vi "test_extended_video.vi"() -> ()   [LabVIEW 2023]
uses:
  <vilib>/picture/picture.llb/Draw True-Color Pixmap.vi
panel:
  in  "profile_index":sgl=4.0
  in  "source_index":sgl=2.0
  in  "group_index":sgl
  out "metadata":T1
  in  "host":string="192.168.1.7"
  in  "path in":path=path "C:/Users/jcds/Documents/GitHub/hl2ss/extensions/client_labview/hl2ss_labview/hl2ss_ulm.dll"
  out "Pose":sgl[][](array[numeric])
  out "Video":picture
  in  "stop":bool
  in  "Framerate":u8=30
  in  "Height":u16=360
  in  "Width":u16=640
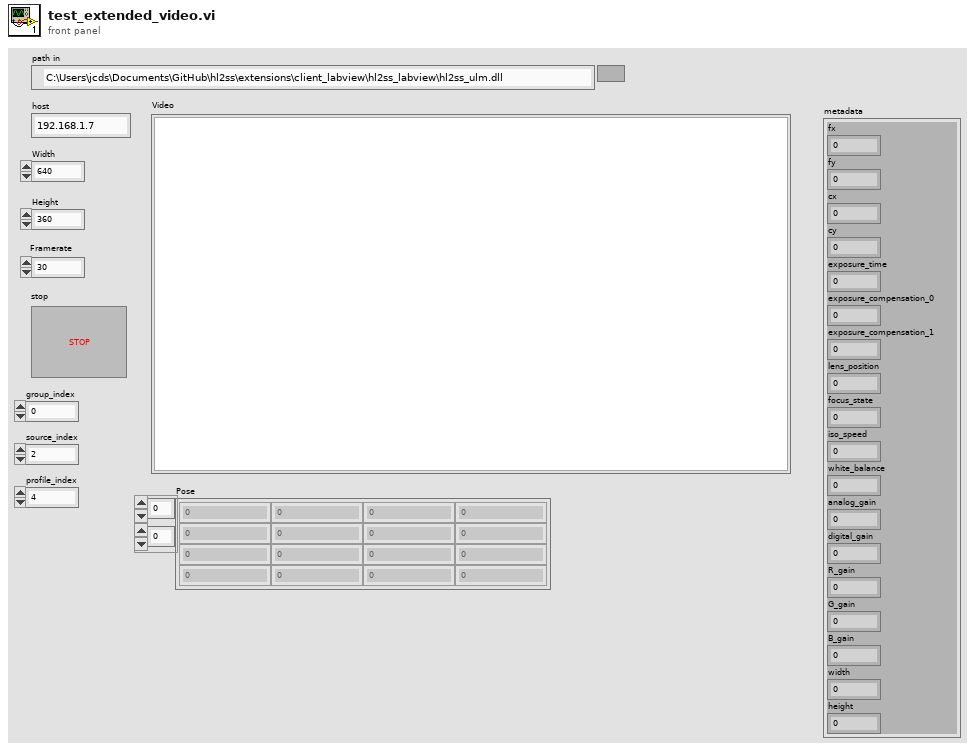
[diagram p1: front panel]
types:
  T1 = cluster{"fx":sgl, "fy":sgl, "cx":sgl, "cy":sgl, "exposure_time":u64, "exposure_compensation_0":u64, "exposure_compensation_1":u64, "lens_position":u32, "focus_state":u32, "iso_speed":u32, "white_balance":u32, "analog_gain":sgl, "digital_gain":sgl, "R_gain":sgl, "G_gain":sgl, "B_gain":sgl, "width":u16, "height":u16}
  T2 = cluster{"enable_mrc":u8, "hologram_composition":u8, "recording_indicator":u8, "video_stabilization":u8, "blank_protected":u8, "show_mesh":u8, "shared":u8, "_reserved_0":u8, "global_opacity":sgl, "output_width":sgl, "output_height":sgl, "video_stabilization_length":u32, "hologram_perspective":u32, "_reserved_1":u32}
  T3 = cluster{"chunk":u64, "mode":u8, "_reserved_0":u8, "width":u16, "height":u16, "framerate":u8, "divisor":u8, "profile":u8, "level":u8, "_reserved_1":u16, "bitrate":u32, "options_size":i64, "options_data":u64, "_reserved_2":u64}
  T4 = cluster{"frame_stamp":i64, "timestamp":u64, "payload_size":u32, "status":i32, "payload":u64, "pose":u64}
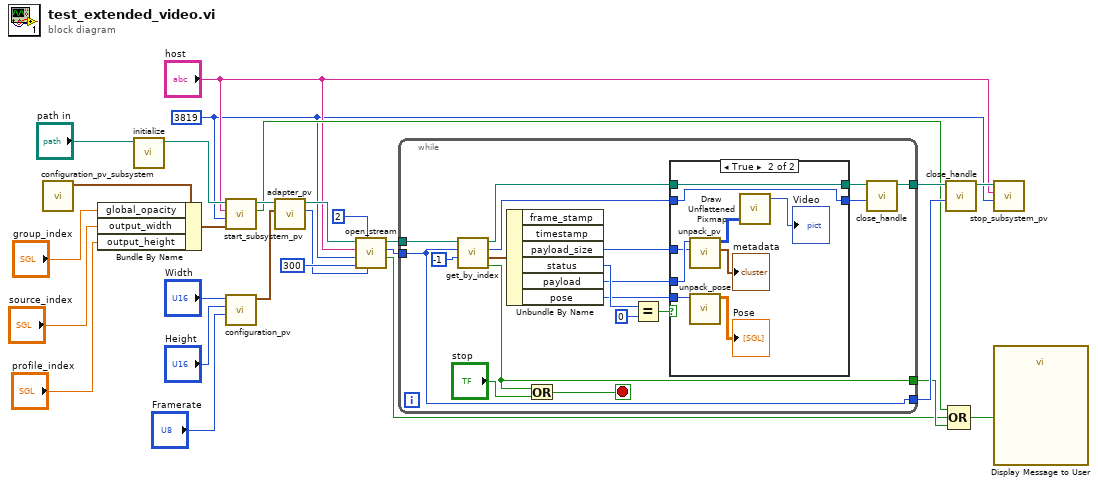
[diagram p0: block diagram]
diagram:
  w7 = u16 3819 ("port")
  n1 = call "configuration_pv_subsystem.vi"() -> ("configuration_pv_subsystem"=w6:T2)  [unwired: 11 in]
  n2 = Bundle By Name(cluster=w6, "global_opacity"="group_index", "output_width"="source_index", "output_height"="profile_index") -> (w5:T2)
  n3 = call "initialize.vi"("path in"="path in") -> ("path out"=w19:path)  [unwired: 9 in, 1 out]
  n4 = call "start_subsystem_pv.vi"("configuration"=w5, "port"=w7, "host"="host", "path in"=w19) -> ("error"=w11:bool, "path out"=w15:path)  [unwired: 6 in]
  n5 = call "configuration_pv.vi"("framerate"="Framerate", "height"="Height", "width"="Width") -> ("configuration_pv"=w14:T3)  [unwired: 8 in]
  n6 = call "adapter_pv.vi"("configuration_pv"=w14, "path in"=w15) -> ("configuration"=w12:u64, "path out"=w13:path)  [unwired: 8 in]
  n7 = call "open_stream.vi"("configuration"=w12, "decoded"=u8 2, "buffer_size"=u64 300, "port"=w7, "host"="host", "path in"=w13) -> ("error"=w9:bool, "handle"=w10:u64, "path out"=w26:path)  [unwired: 3 in]
  n8 = while {
    tunnel: w10 -> [w35]
    tunnel: w26 -> [w43]
    tunnel: [w35] -> w25
    tunnel: [w34] -> w24
    tunnel: [w31] -> w21
    stop <- w44 stop-if-true
    n9 = call "get_by_index.vi"("frame_stamp"=i64 -1, "stream_handle"=w35, "path in"=w43) -> ("error"=w31:bool, "packet"=w32:T4, "packet_handle"=w33:u64, "path out"=w29:path)  [unwired: 5 in]
    n10 = Unbundle By Name(w32) -> ("payload_size"=w28:u32, "status"=w38:i32, "payload"=w37:u64, "pose"=w36:u64)  [unwired: 2 out]
    n11 = Or(x=w31, y="stop") -> (x .or. y?=w44:bool)
    n12 = Equal?(x=w38, y=0) -> (x = y?=w40:bool)
    n13 = case shown="True" w40 {
      tunnel: [w47 w56] -> w39
      tunnel: w33 -> [w47 w56]
      tunnel: w37 -> [_ w52]
      tunnel: w36 -> [_ w53]
      tunnel: [w46 w49] -> w30
      tunnel: w29 -> [w46 w49]
      tunnel: w28 -> [_ w48]
      frame False {
      }
      frame True {
        n14 = call "unpack_pv.vi"("payload_size"=w48, "payload"=w52) -> ("metadata"=→"metadata":T1, "image"=w51:u32[][])  [unwired: 5 in, 3 out]
        n15 = call "unpack_pose.vi"("pose"=w53) -> ("pose"=→"Pose":sgl[][])  [unwired: 9 in, 1 out]
        n16 = call-poly <vilib>:"Draw Unflattened Pixmap.vi"("data (RGB format)"=w51) -> ("new picture"=→"Video":picture)  [unwired: 8 in]
      }
    }
    n17 = call "close_handle.vi"("handle"=w39, "path in"=w30) -> ("path out"=w34:path)  [unwired: 9 in]
  }
  n18 = call "close_handle.vi"("handle"=w25, "path in"=w24) -> ("path out"=w23:path)  [unwired: 9 in]
  n19 = Compound Arithmetic op=OR(w11, w9, w21) -> (w22:bool)
  n20 = call "stop_subsystem_pv.vi"("port"=w7, "host"="host", "path in"=w23) -> ()  [unwired: 7 in, 2 out]
  n21 = call "Display Message to User"("Enable"=w22) -> ()  [unwired: 9 in, 2 out]
